vi "WriteDatalogSubVI.vi"(11 "VI in":refnum<vi>) -> ()   [LabVIEW 2019]
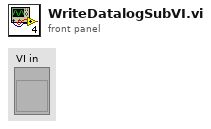
[diagram p1: front panel]
types:
  T1 = enum16{"open", "replace", "create", "open or create", "replace or create", "replace or create with confirmation"}
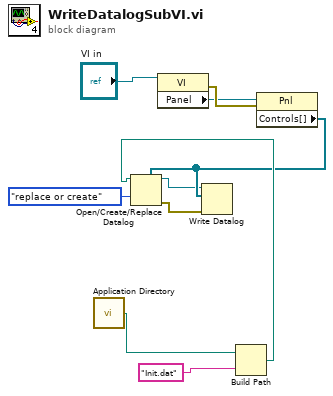
[diagram p0: block diagram]
diagram:
  n1 = call <vilib>:"Application Directory.vi"() -> ("Application Directory"=w10:path)
  n2 = property class="VI"(reference="VI in") -> (error out=w4:errorcluster, "Panel"=w3:refnum<vi>)  [unwired: 1 in, 1 out]
  n3 = Build Path(base path=w10, name or relative path="Init.dat") -> (appended path=w9:path)
  n4 = property class="Pnl"(reference=w3, error in=w4) -> ("Controls[]"=w7:refnum<vi>[])  [unwired: 2 out]
  n5 = Open/Create/Replace Datalog(5:w7, 10:T1."replace or create" ("operation (0:open)"), 11:w9) -> (0:w6:errorcluster, 3:w5:refnum<k1>)  [unwired: 3 in, 1 out]
  n6 = Write Datalog(4:w6, 6:w7, 7:w5) -> ()  [unwired: 2 out]
